vi "RR autofocus calibrate.vi"(8 "error in":errorcluster) -> (0 "error out":errorcluster, 2 "Intensity OK":bool=TRUE, 3 "Cal. curve":cluster{ext[], dbl[]})   [LabVIEW 2011]
doc: "Aquires a z-stack of images, calculates the goodness-of-focus (GOF) parameter for each image, and returns the stage to the z position with max GOF. Parameters of the autofocusing process are set (and can be adjusted during acquisition) using the Autofocus Globals.vi front panel."
uses:
  Stage/Move stage command.ctl
  Autofocus Globals.vi
  h-nu shutters/hardware status globals.vi
panel:
  out "Calibration curve":cluster{ext[], dbl[]}(graph)
  # "not for interactive use"
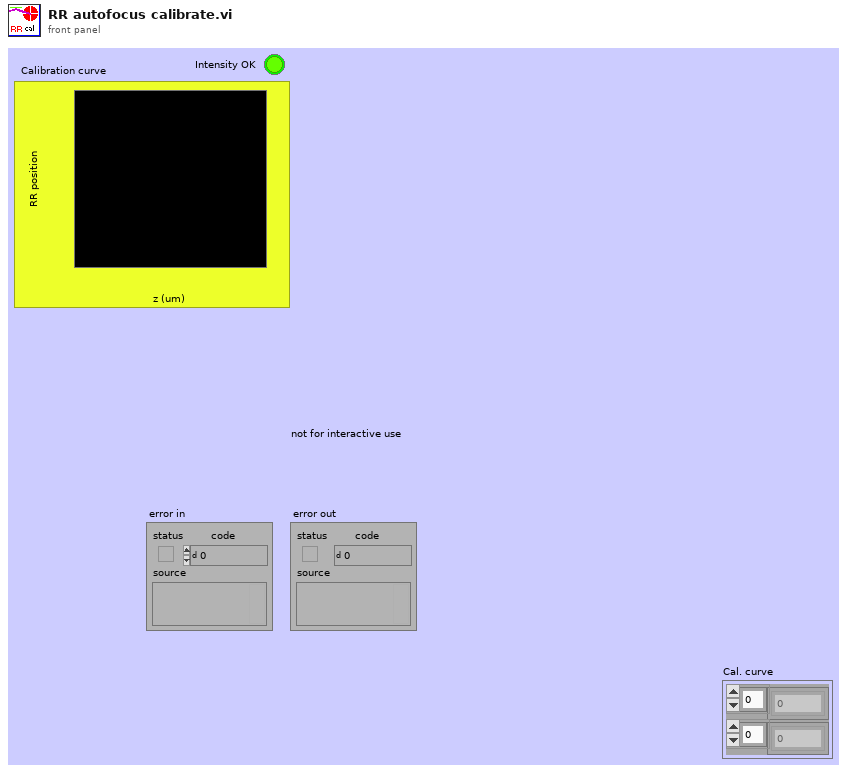
[diagram p1: front panel]
types:
  T1 = typedef "Move stage command.ctl" = cluster{"dx (um) (0 -> ignore)":ext, "dy (um) (0 -> ignore)":ext, "dz (um) (0 -> ignore)":ext, "Re-center x,y":bool, "Re-center z":bool, "x (um) (-1 -> ignore)":dbl, "y (um) (-1 -> ignore)":dbl, "z (um) (-1 -> ignore)":dbl}
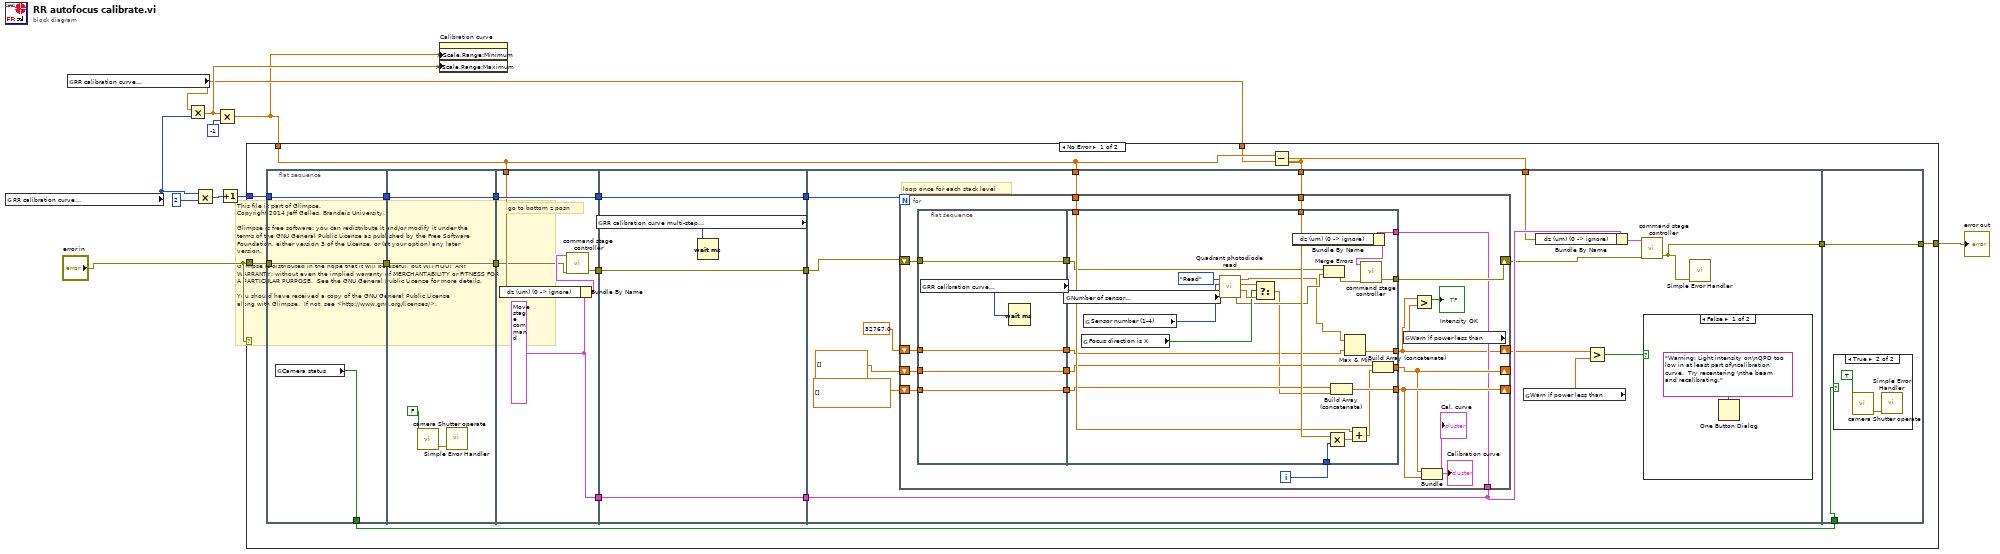
[diagram p0: block diagram]
diagram:
  # "This file is part of Glimpse. \nCopyright 2014 Jeff Gelles, Brandeis University.    \n\nGlimpse is free software: you can redistribute it and/or modify it under the \nterms of the GNU General Public License as published by the Free Software \nFoundation, either version 3 of the License, or (at your option) any later \nversion.\n\nGlimpse is distributed in the hope that it will be useful, but WITHOUT ANY \nWARRANTY; without even the implied warranty of MERCHANTABILITY or FITNESS FOR \nA PARTICULAR PURPOSE.  See the GNU General Public License for more details.\n\nYou should have received a copy of the GNU General Public License\nalong with Glimpse.  If not, see <http://www.gnu.org/licenses/>."
  n1 = global read "Autofocus Globals.vi" "RR calibration curve\nhalf-width  (steps)"() -> (w6:u16)
  n2 = global read "Autofocus Globals.vi" "RR calibration curve\nstep size (um)"() -> (w4:ext)
  n3 = Multiply(x=w4, y=w6) -> (x*y=w5:ext)
  n4 = Multiply(x=w6, y=i16 2) -> (x*y=w9:u16)
  n5 = Multiply(x=w5, y=i16 -1) -> (x*y=w3:ext)
  n6 = Increment(x=w9) -> (x+1=w7:u16)
  n7 = case shown="No Error" "error in" {
    selector: "error in" -> [_ w115]
    tunnel: w7 -> [w22 _]
    tunnel: w4 -> [w17 _]
    tunnel: w3 -> [w18 _]
    tunnel: "error in" -> [w21 _]
    tunnel: [w20 w115] -> w2
    frame No Error {
      n8 = flat-sequence {
        tunnel: w21 -> [w30]
        tunnel: w22 -> [w31]
        tunnel: [w31] -> w14
        tunnel: [w30] -> w13
        tunnel: [w29] -> w11
        tunnel: [w35] -> w16
        tunnel: [w34] -> w15
        tunnel: w14 -> [w35]
        tunnel: w13 -> [w34]
        tunnel: [w41] -> w28
        tunnel: w18 -> [w38]
        tunnel: [w39] -> w27
        tunnel: [w37] -> w26
        tunnel: w16 -> [w41]
        tunnel: w15 -> [w36]
        tunnel: w28 -> [w45]
        tunnel: [w45] -> w25
        tunnel: w27 -> [w44]
        tunnel: [w44] -> w24
        tunnel: [w42] -> w23
        tunnel: w26 -> [w42]
        tunnel: w25 -> [w60]
        tunnel: w24 -> [w53]
        tunnel: w17 -> [w59]
        tunnel: w18 -> [w57]
        tunnel: w23 -> [w54]
        tunnel: w19 -> [w50]
        tunnel: [w47] -> w12
        tunnel: [w112] -> w20
        tunnel: w12 -> [w112]
        tunnel: w11 -> [w111]
        frame #0 {
          n9 = global read "hardware status globals.vi" "Camera status"() -> (w29:bool)
        }
        frame #1 {
          n10 = call "camera Shutter operate.vi"("Open?"=FALSE) -> ("error out"=w32:errorcluster)  [unwired: 1 in, 6 out]
          n11 = call <vilib>:"Simple Error Handler.vi"("error in (no error)"=w32) -> ()  [unwired: 1 in, 8 out]
        }
        frame #2 {
          w37 = T1 {"dx (um) (0 -> ignore)"=0.0, "dy (um) (0 -> ignore)"=0.0, "dz (um) (0 -> ignore)"=0.0, "Re-center x,y"=FALSE, "Re-center z"=FALSE, "x (um) (-1 -> ignore)"=-1.0, "y (um) (-1 -> ignore)"=-1.0, "z (um) (-1 -> ignore)"=-1.0} ("command")
          # "go to bottom z posn"
          n12 = Bundle By Name(cluster=w37, "dz (um) (0 -> ignore)"=w38) -> (w40:T1)
          n13 = call "command stage controller.vi"("command"=w40, "error in (no error)"=w36) -> ("error out"=w39:errorcluster)  [unwired: 6 out]
        }
        frame #3 {
          n14 = global read "Autofocus Globals.vi" "RR calibration curve multi-step\nadd'l settle time (ms)"() -> (w43:u16)
          n15 = Wait (ms)(milliseconds to wait=w43) -> ()  [unwired: 1 out]
        }
        frame #4 {
          # "loop once for each stack level"
          n16 = for {
            N: w60 -> [_]
            shift-right: [w77] -> w48
            shift-left: w53 -> [w79]
            tunnel: w59 -> [w78]
            shift-right: [w69] -> _
            shift-left: dbl[] [] ("QPD position") -> [w76]
            shift-right: [w68] -> _
            shift-left: dbl[] [] ("z (um)") -> [w71]
            tunnel: w57 -> [w73]
            tunnel: w54 -> [w67]
            shift-right: [w62] -> w51
            shift-left: 32767.0 -> [w65]
            i -> [w74]
            n17 = flat-sequence {
              tunnel: w79 -> [w84]
              tunnel: [w84] -> w80
              tunnel: w76 -> [w83]
              tunnel: [w83] -> w75
              tunnel: [w82] -> w72
              tunnel: w71 -> [w82]
              tunnel: [w81] -> w66
              tunnel: w65 -> [w81]
              tunnel: w80 -> [w95]
              tunnel: w78 -> [w106]
              tunnel: [w109] -> w77
              tunnel: [w108] -> w69
              tunnel: w75 -> [w98]
              tunnel: w74 -> [w107]
              tunnel: w73 -> [w104]
              tunnel: w72 -> [w97]
              tunnel: [w103] -> w68
              tunnel: w67 -> [w101]
              tunnel: [w88] -> w62
              tunnel: w66 -> [w87]
              frame #0 {
                n18 = global read "Autofocus Globals.vi" "RR calibration curve\nsettle time (ms)"() -> (w85:u16)
                n19 = Wait (ms)(milliseconds to wait=w85) -> ()  [unwired: 1 out]
              }
              frame #1 {
                n20 = global read "Autofocus Globals.vi" "Number of sensor\nreadings to average"() -> (w86:i32)
                n21 = global read "Autofocus Globals.vi" "Focus direction is X"() -> (w92:bool)
                n22 = global read "Autofocus Globals.vi" "Sensor number (1-4)"() -> (w99:i8)
                n23 = call "Quadrant photodiode read.vi"("Sensor Number\n(ignored)"=w99, "number of readings\n to average"=w86, "Mode"=enum16{"Start", "Read", "End"}."Read") -> ("error out"=w91:errorcluster, "Y position"=w93:dbl, "X position"=w94:dbl, "Power"=w89:dbl)  [unwired: 3 out]
                n24 = Select(t=w94, s=w92, f=w93) -> (s? t:f=w90:dbl)
                n25 = Bundle By Name(cluster=w101, "dz (um) (0 -> ignore)"=w106) -> (w110:T1)
                n26 = Merge Errors(w95, w91) -> (w96:errorcluster)
                n27 = Multiply(x=w106, y=w107) -> (x*y=w105:ext)
                n28 = Build Array (concatenate)(w98, w90) -> (w108:dbl[])
                n29 = Max & Min(x=w89, y=w87) -> (min(x,y)=w88:dbl)  [unwired: 1 out]
                n30 = Add(x=w104, y=w105) -> (x+y=w102:ext)
                n31 = call "command stage controller.vi"("command"=w110, "error in (no error)"=w96) -> ("error out"=w109:errorcluster)  [unwired: 6 out]
                n32 = Build Array (concatenate)(w97, w102) -> (w103:ext[])
              }
            }
            n33 = global read "Autofocus Globals.vi" "Warn if power less than"() -> (w64:dbl)
            n34 = Greater?(x=w62, y=w64) -> (0:→"Intensity OK":bool)
            n35 = Bundle(w68, w69) -> (→"Calibration curve" →"Cal. curve":cluster{ext[], dbl[]})  [unwired: 1 out]
          }
          n36 = global read "Autofocus Globals.vi" "Warn if power less than"() -> (w56:dbl)
          n37 = Bundle By Name(cluster=w54, "dz (um) (0 -> ignore)"=w50) -> (w49:T1)
          n38 = Greater?(x=w51, y=w56) -> (0:w55:bool)
          n39 = call "command stage controller.vi"("command"=w49, "error in (no error)"=w48) -> ("error out"=w47:errorcluster)  [unwired: 6 out]
          n40 = case shown="False" w55 {
            frame False {
              n41 = One Button Dialog(message="Warning: Light intensity on\nQPD too low in at least part of\ncalibration curve.  Try recentering \nthe beam and recalibrating.") -> ()  [unwired: 2 out]
            }
            frame True {
            }
          }
          n42 = call <vilib>:"Simple Error Handler.vi"("error in (no error)"=w47) -> ()  [unwired: 1 in, 8 out]
        }
        frame #5 {
          n43 = case shown="True" w111 {
            frame False {
            }
            frame True {
              n44 = call "camera Shutter operate.vi"("Open?"=TRUE) -> ("error out"=w113:errorcluster)  [unwired: 1 in, 6 out]
              n45 = call <vilib>:"Simple Error Handler.vi"("error in (no error)"=w113) -> ()  [unwired: 1 in, 8 out]
            }
          }
        }
      }
      n46 = Subtract(x=w18, y=w17) -> (x-y=w19:ext)
    }
    frame Error {
    }
  }
  "error out" <- w2
  n47 = property on="Calibration curve" class="XYGraph (strict)"("X Scale.Range:Minimum"=w3, "X Scale.Range:Maximum"=w5) -> ()  [unwired: 2 in, 2 out]
